vi "3-integer 8bit result.vi"() -> ()   [LabVIEW 2018]
panel:
  out "Product":i8
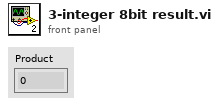
[diagram p1: front panel]
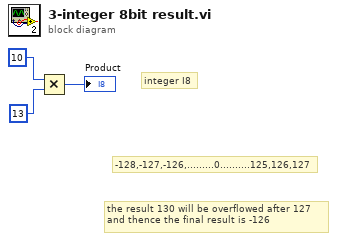
[diagram p0: block diagram]
diagram:
  # "the result 130 will be overflowed after 127 \nand thence the final result is -126"
  # "-128,-127,-126,.........0..........125,126,127"
  # "integer I8"
  n1 = Multiply(x=i8 10, y=i8 13) -> (x*y=→"Product":i8)
